vi "Corect Pressure Block.vi"(0 "U in":dbl format="%#_13g", 5 "SP [MPa]":dbl format="%#_13g", 7 "PV [MPa]":dbl format="%#_13g", 12 "delta":dbl, 13 "MPa per Volt":dbl) -> (4 "U out":dbl format="%#_13g")   [LabVIEW 2019]
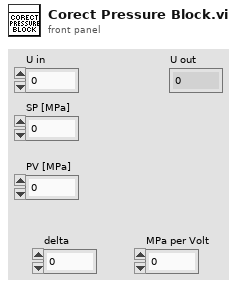
[diagram p1: front panel]
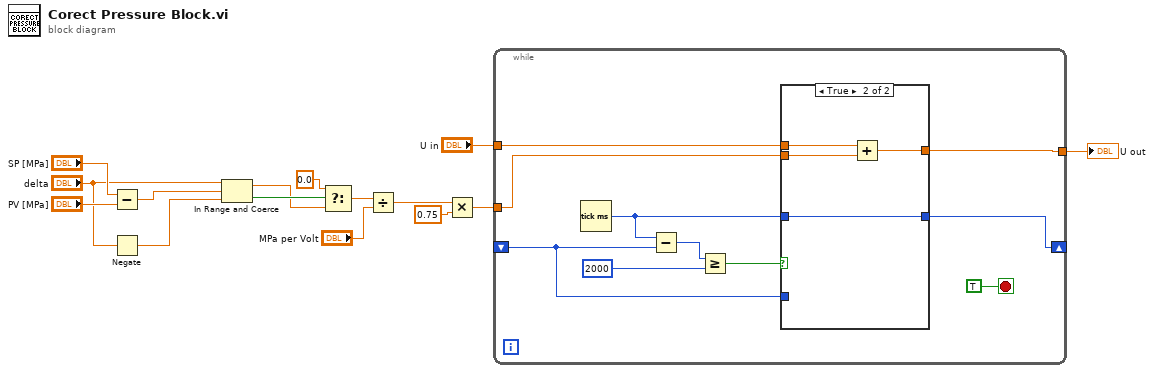
[diagram p0: block diagram]
diagram:
  n1 = Subtract(x="SP [MPa]", y="PV [MPa]") -> (x-y=w4:dbl)
  n2 = Negate(x="delta") -> (-x=w8:dbl)
  n3 = In Range and Coerce(upper limit="delta", x=w4, lower limit=w8) -> (coerced(x)=w3:dbl, In Range?=w6:bool)
  n4 = Select(t=0.0, s=w6, f=w3) -> (s? t:f=w2:dbl)
  n5 = Divide(x=w2, y="MPa per Volt") -> (x/y=w1:dbl)
  n6 = Multiply(x=w1, y=0.75) -> (x*y=w11:dbl)
  n7 = while {
    tunnel: w11 -> [w23]
    tunnel: "U in" -> [w24]
    tunnel: [w22] -> w9
    shift-right: [w21] -> _
    shift-left: _ -> [w16]
    stop <- TRUE stop-if-true
    n8 = Tick Count (ms)() -> (millisecond timer value=w20:u32)
    n9 = Subtract(x=w20, y=w16) -> (x-y=w19:u32)
    n10 = Greater Or Equal?(x=w19, y=u32 2000) -> (x >= y?=w17:bool)
    n11 = case shown="True" w17 {
      tunnel: w24 -> [w27 w31]
      tunnel: w23 -> [_ w30]
      tunnel: [w27 w29] -> w22
      tunnel: [w26 w28] -> w21
      tunnel: w20 -> [_ w28]
      tunnel: w16 -> [w26 _]
      frame False {
      }
      frame True {
        n12 = Add(x=w31, y=w30) -> (x+y=w29:dbl)
      }
    }
  }
  "U out" <- w9
